vi "Base Construct.vi"(6 "channels":u8[](array[numeric]), 8 "error in":errorcluster, 9 "hardware handles":T1, 10 "identifier":string, 11 "execution unit in":refnum<class "Execution Unit.lvclass">) -> (0 "error out":errorcluster, 3 "execution unit out":refnum<class "Execution Unit.lvclass">)   [LabVIEW 2020, in "AIM ARINC 429 Engine.lvlib" / "Implementation.lvlib" / "Execution Unit.lvclass"]
uses:
  Execution Unit.lvclass
  Custom Device/Hardware Handles.ctl
  Custom Device/Custom Device.lvlib
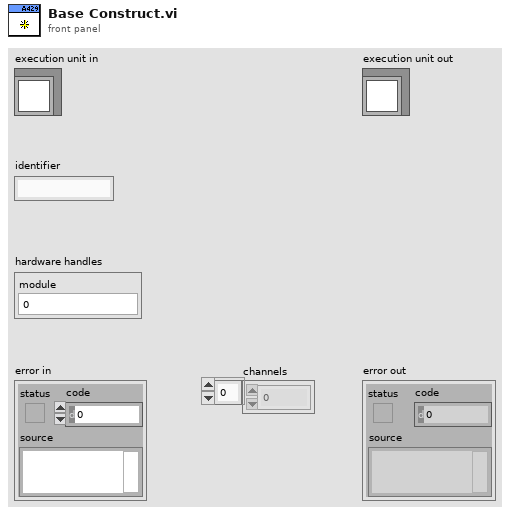
[diagram p1: front panel]
types:
  T1 = typedef "AIM ARINC 429 Engine.lvlib/Custom Device.lvlib/Hardware Handles.ctl" = cluster{"module":u8}
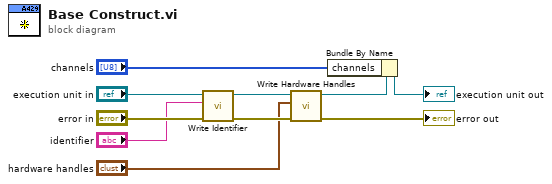
[diagram p0: block diagram]
diagram:
  n1 = call "Write Identifier.vi"("error in (no error)"="error in", "identifier"="identifier", "Ballard ARINC-429 Execution Unit in"="execution unit in") -> ("error out"=w8:errorcluster, "Ballard ARINC-429 Execution Unit out"=w9:refnum<class "Execution Unit.lvclass">)  [unwired: 7 in]
  n2 = call "Write Hardware Handles.vi"("error in"=w8, "hardware handles"="hardware handles", "AIM ARINC-429 execution unit in"=w9) -> ("error out"=→"error out":errorcluster, "AIM ARINC-429 execution unit out"=w7:refnum<class "Execution Unit.lvclass">)  [unwired: 7 in]
  n3 = Bundle By Name(cluster=w7, "channels"="channels") -> (→"execution unit out":refnum<class "Execution Unit.lvclass">)
